vi "Shift Register Cell.vi"(8 "load":bool, 9 "shift":bool, 10 "Rxy shift":u64, 11 "Rxy load":u64) -> (3 "Rxy":u64)   [LabVIEW 2017]
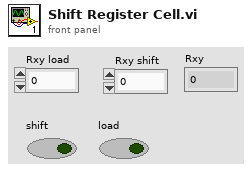
[diagram p1: front panel]
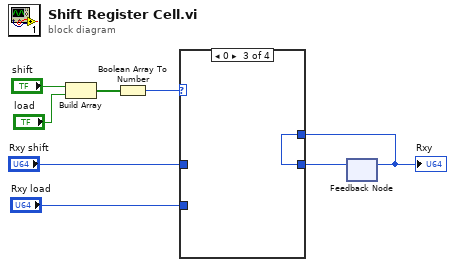
[diagram p0: block diagram]
diagram:
  n1 = Build Array("shift", "load") -> (w6:bool[])
  n2 = Boolean Array To Number(Boolean array=w6) -> (number=w5:u32)
  n3 = feedback #1() -> (w1:u64)  [unwired: 1 in]
  "Rxy" <- w1
  n4 = case shown="0" w5 {
    tunnel: "Rxy shift" -> [_ _ _ w12]
    tunnel: "Rxy load" -> [w9 w10 _ _]
    tunnel: [w9 w10 w11 w12] -> w2
    tunnel: w1 -> [_ _ w11 _]
    frame 2 {
    }
    frame 3 {
    }
    frame 0 {
    }
    frame 1, Default {
    }
  }
  n5 = feedback-in #1(w2) -> ()
